vi "Test Namer with Shared Approval File Decorating Namer with Folder.vi"   [LabVIEW 2020, in "Namer.Tests.lvclass"]
uses:
  Namer.Tests.lvclass
  Source/Approval Tests/Namer with Folder/Namer with Folder.lvclass
  C:/Users/ImageBuilderAdmin/Desktop/ApprovalTests.LabVIEW/Source/Approval Tests/Namer/Namer.lvclass
  Source/Approval Tests/Naming Data/Naming Data.lvclass
  Source/Approval Tests/Namer With Shared Approved File/Namer With Shared Approved File.lvclass
  C:/Users/ImageBuilderAdmin/Desktop/ApprovalTests.LabVIEW/Source/Approval Tests/Namer Decorator/Namer Decorator.lvclass
  Source/Approval Tests/Naming Data/Naming Data.lvclass/Naming Data.ctl
  Source/Approval Tests/Namer With Shared Approved File/Namer With Shared Approved File.lvclass/Namer With Shared Approved File.ctl
  Source/Approval Tests/Namer Decorator/Namer Decorator.lvclass/Namer Decorator.ctl
  <vilib>/addons/_JKI Toolkits/Caraya/classes/Test/Test.lvclass
  <vilib>/addons/_JKI Toolkits/Caraya/classes/Assert/Assert.lvclass
  <vilib>/addons/_JKI Toolkits/Caraya/classes/Assert/Assert Equal Value and Type_Variant.vi
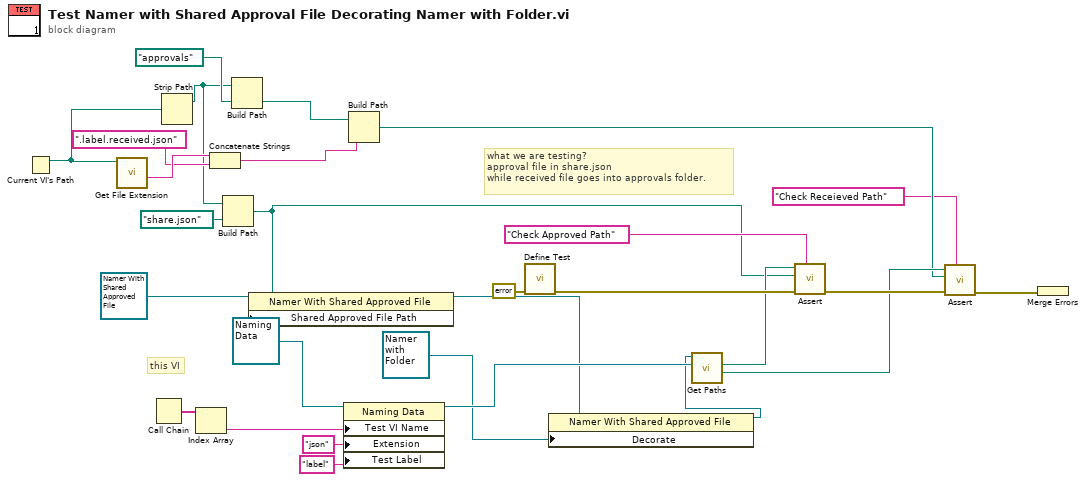
[diagram p0: block diagram]
diagram:
  # "what we are testing?\napproval file in share.json\nwhile received file goes into approvals folder."
  # "this VI"
  n1 = Current VI's Path() -> (path=w17:path)
  n2 = call <vilib>:"Get File Extension.vi"("file"=w17) -> ("filename without extension"=w16:string)  [unwired: 6 in, 4 out]
  n3 = Call Chain() -> (call chain=w24:string[])
  n4 = Strip Path(path=w17) -> (stripped path=w3:path)  [unwired: 1 out]
  n5 = Index Array(array=w24) -> (element=w23:string)  [unwired: 1 in]
  n6 = Concatenate Strings(w16, ".label.received.json" ("string")) -> (w14:string)
  n7 = Build Path(base path=w3, name or relative path=path "share.json") -> (appended path=w1:path)
  n8 = Build Path(base path=w3, name or relative path=path "approvals") -> (appended path=w9:path)
  n9 = property class="Namer With Shared Approved File"(reference=refnum<class "Namer With Shared Approved File.lvclass"> refnum ("Approval Tests:Namer With Shared Approved File.lvclass"), "Shared Approved File Path"=w1) -> (reference out=w4:refnum<class "Namer With Shared Approved File.lvclass">)  [unwired: 1 in, 1 out]
  n10 = property on="Property Node" class="Naming Data"(reference=refnum<class "Naming Data.lvclass"> refnum ("Naming Data"), "Test VI Name"=w23, "Extension"="json", "Test Label"="label") -> (reference out=w22:refnum<class "Naming Data.lvclass">)  [unwired: 1 in, 1 out]
  n11 = Build Path(base path=w9, name or relative path=w14) -> (appended path=w13:path)
  n12 = call <vilib>:"Define Test.vi"("error in (no error)"=errorcluster {"status"=FALSE, "code"=0, "source"=""}) -> ("error out"=w27:errorcluster)  [unwired: 9 in, 1 out]
  n13 = property class="Namer With Shared Approved File"(reference=w4, "Decorate"=refnum<class "Namer with Folder.lvclass"> refnum ("Approval Tests:Namer with SubFolder.lvclass")) -> (reference out=w5:refnum<class "Namer With Shared Approved File.lvclass">)  [unwired: 1 in, 1 out]
  n14 = call-dynamic "Get Paths.vi"("Naming Data"=w22, "Namer With Shared Approved File in"=w5) -> ("Received Path"=w18:path, "Approved Path"=w19:path)  [unwired: 6 in, 2 out]
  n15 = call-poly <vilib>:"Assert.vi"("Label"="Check Approved Path" ("Label (VI Title)"), "error in (no error)"=w27, "Actual"=w1, "Expected"=w19) -> ("error out"=w21:errorcluster)  [unwired: 6 in, 1 out]
  n16 = call-poly <vilib>:"Assert.vi"("Label"="Check Receieved Path" ("Label (VI Title)"), "error in (no error)"=w21, "Actual"=w13, "Expected"=w18) -> ("error out"=w20:errorcluster)  [unwired: 6 in, 1 out]
  n17 = Merge Errors(w20) -> ()  [unwired: 1 out]
